vi "LV10_7.vi"() -> ()   [LabVIEW 2016]
uses:
  <vilib>/picture/picture.llb/Draw 8-Bit Pixmap.vi
  <vilib>/imath/engines/lvmath2/RunTimeEngine/BuiltInFunctions/randnormal/NIMS_randnormal(Str,I32).vi
  <vilib>/imathl/engines/lvmath/Functions/Error Handling/Create Error.vi
  <vilib>/imath/engines/lvmath2/RunTimeEngine/BuiltInFunctions/randnormal/NIMS_randnormal(I32,I32).vi
  <vilib>/imath/engines/lvmath2/RunTimeEngine/BuiltInFunctions/fft2d/NIMS_fft2d.vi
  <instcachedir>/0/NIMS_fft2d_01A33FFC48FF4786A19C9A8A715D9BC4.lvgen/NIMS_fft2d_01A33FFC48FF4786A19C9A8A715D9BC4_000.vi
  <vilib>/imath/engines/lvmath2/RunTimeEngine/BuiltInFunctions/abs/NIMS_abs(signed).vi
  <instcachedir>/0/NIMS_abs(signed)_C4FCB8E6058B49B797C7C8D53CA5F6EC.lvgen/NIMS_abs(signed)_C4FCB8E6058B49B797C7C8D53CA5F6EC_003.vi
  <vilib>/imath/engines/lvmath2/RunTimeEngine/BuiltInFunctions/findnz/NIMS_[1o]_findnz(GM).vi
  <instcachedir>/0/NIMS_[1o]_findnz(GM)_0B85F0C1FD7A4D70A7D15487030BA0C8.lvgen/NIMS_[1o]_findnz(GM)_0B85F0C1FD7A4D70A7D15487030BA0C8_004.vi
  <vilib>/imath/engines/lvmath2/RunTimeEngine/ErrorHandling/NIMS_Error From Error Code.vi
  <vilib>/imath/engines/lvmath2/RunTimeEngine/IndexReplace/NIMS M(S,S)=S.vi
  <instcachedir>/0/NIMS M(S,S)=S_98E40400474E4398B113AE20298B4F82.lvgen/NIMS M(S,S)=S_98E40400474E4398B113AE20298B4F82_002.vi
  <vilib>/imath/engines/lvmath2/RunTimeEngine/IndexRead/NIMS M(M).vi
  <instcachedir>/0/NIMS M(M)_EB00EBD471DD47B0915ED9997EB5A993.lvgen/NIMS M(M)_EB00EBD471DD47B0915ED9997EB5A993_004.vi
  <vilib>/imath/engines/lvmath2/RunTimeEngine/IndexReplace/NIMS M(M)=M.vi
  <instcachedir>/0/NIMS M(M)=M_D07272DCF1984374AF2B42254FCB82DF.lvgen/NIMS M(M)=M_D07272DCF1984374AF2B42254FCB82DF_003.vi
  <vilib>/imath/engines/lvmath2/RunTimeEngine/ErrorHandling/NIMS_Create Error From Enums.vi
  <vilib>/imath/engines/lvmath2/RunTimeEngine/BuiltInFunctions/norm/NIMS_norm(GV,DBL).vi
  <instcachedir>/0/NIMS_norm(GV,DBL)_1268AFF3C646412B8C6EA3CE75D09042.lvgen/NIMS_norm(GV,DBL)_1268AFF3C646412B8C6EA3CE75D09042_000.vi
  <vilib>/imath/engines/lvmath2/RunTimeEngine/BuiltInFunctions/length/NIMS_length(GV).vi
  <instcachedir>/0/NIMS_length(GV)_08A3D13377FD4E4B96F5795FBF3698FA.lvgen/NIMS_length(GV)_08A3D13377FD4E4B96F5795FBF3698FA_000.vi
  <vilib>/imath/engines/lvmath2/RunTimeEngine/BuiltInFunctions/mirrorh/NIMS_mirrorh(GRowV).vi
  <instcachedir>/0/NIMS_mirrorh(GRowV)_B6A8CC4EAFBA4F9A82A59460D67BDFF0.lvgen/NIMS_mirrorh(GRowV)_B6A8CC4EAFBA4F9A82A59460D67BDFF0_000.vi
  <vilib>/imath/engines/lvmath2/RunTimeEngine/RangeToken/NIMS_Range.vi
  <instcachedir>/0/NIMS_Range_A7C094595B484CA7AF10685B02D808ED.lvgen/NIMS_Range_A7C094595B484CA7AF10685B02D808ED_001.vi
  <vilib>/imath/engines/lvmath2/RunTimeEngine/ArithmeticOperatorToken/NIMS_ArithmeticOperator_times.vi
  <instcachedir>/0/NIMS_ArithmeticOperator_times_953B34F74CAC448FB707D816A29CC5F0.lvgen/NIMS_ArithmeticOperator_times_953B34F74CAC448FB707D816A29CC5F0_000.vi
  <vilib>/imath/engines/lvmath2/RunTimeEngine/NodeEndStatement/NIMS_NodeEndStatement_Output.vi
  <instcachedir>/0/NIMS_NodeEndStatement_Output_53EC0D466D134D7ABD903AC30B43404B.lvgen/NIMS_NodeEndStatement_Output_53EC0D466D134D7ABD903AC30B43404B_002.vi
  <instcachedir>/0/NIMS_NodeEndStatement_Output_53EC0D466D134D7ABD903AC30B43404B.lvgen/NIMS_NodeEndStatement_Output_53EC0D466D134D7ABD903AC30B43404B_011.vi
  <instcachedir>/0/NIMS_NodeEndStatement_Output_53EC0D466D134D7ABD903AC30B43404B.lvgen/NIMS_NodeEndStatement_Output_53EC0D466D134D7ABD903AC30B43404B_005.vi
  <vilib>/imath/engines/lvmath2/RunTimeEngine/ErrorHandling/NIMS_Finalize Error.vi
panel:
  in  "Threshold l for shrinking":dbl(slide)=0.01 scale=0.001..0.1
  out "Known pixel percentage":dbl=50.43
  out "Original image":picture
  out "Deteriorated image":picture
  in  "Missing pixel density":dbl(slide)=166.0 scale=100.0..200.0
  in  "Max iterations":i32(slide)=98 scale=1.0..500.0
  out "Iterations":i32(slide)=31 scale=-1.0..500.0
  out "Reconstructed image":picture
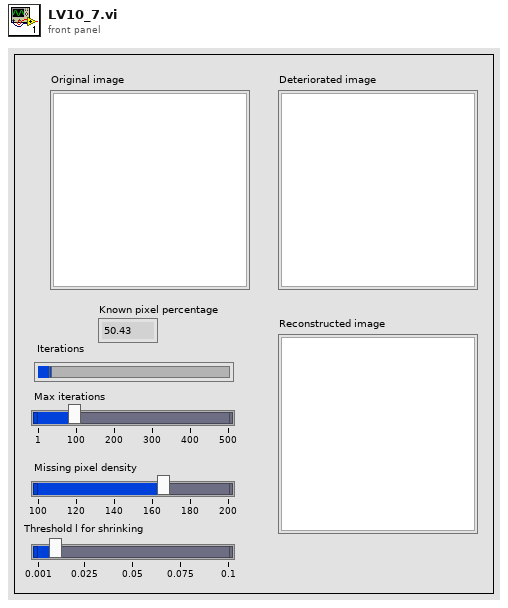
[diagram p1: front panel]
types:
  T1 = typedef "imagedata.ctl" = cluster{"image type":i32, "image depth":i32, "image":u8[], "mask":u8[], "colors":u32[], "Rectangle":cluster{"left":i16, "top":i16, "right":i16, "bottom":i16}}
  T2 = cluster{"ZLL1":dbl[][], "ZLL2":dbl[][], "ZLL3":dbl[][], "ZLH1":dbl[][], "ZLH2":dbl[][], "ZLH3":dbl[][], "ZHL1":dbl[][], "ZHL2":dbl[][], "ZHL3":dbl[][], "ZHH1":dbl[][], "ZHH2":dbl[][], "ZHH3":dbl[][]}
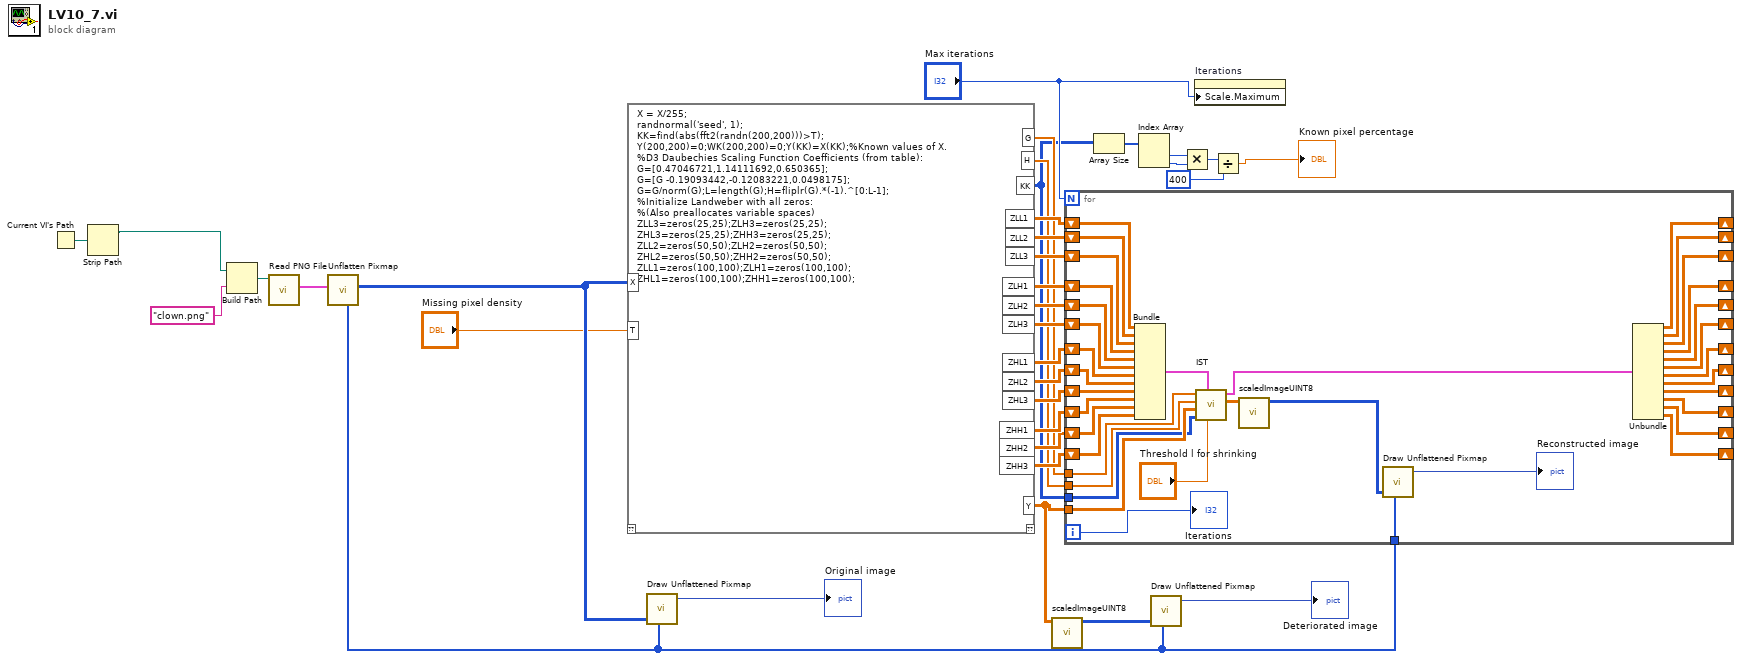
[diagram p0: block diagram]
diagram:
  n1 = Current VI's Path() -> (path=w34:path)
  n2 = Strip Path(path=w34) -> (stripped path=w1:path)  [unwired: 1 out]
  n3 = Build Path(base path=w1, name or relative path="clown.png") -> (appended path=w32:path)
  n4 = call <vilib>:"Read PNG File.vi"("path to PNG file"=w32) -> ("image data"=w31:T1)  [unwired: 8 in, 2 out]
  n5 = call <vilib>:"Unflatten Pixmap.vi"("image data"=w31) -> ("8-bit pixmap"=w29:u8[][], "colors"=w30:u32[])  [unwired: 4 in, 5 out]
  n6 = mathscript code="X = X/255;\nrandnormal('seed', 1);\nKK=find(abs(fft2(randn(200,200)))>T);\nY(200,200)=0;WK(200,200)=0;Y(KK)=X(KK);%Known values of X.\n%D3 Daubechies Scaling Function Coefficients (from table):\nG=[0.47046721,1.14111692,0.650365];\nG=[G -0.19093442,-0.12083221,0.0498175];\nG=G/norm(G);L=length(G);H=fliplr(G).*(-1).^[0:L-1];\n%Initialize Landweber with all zeros:\n%(Also preallocates variable spaces)\nZLL3=zeros(25,25);ZLH3=zeros(25,25);\nZHL3=zeros(25,25);ZHH3=zeros(25,25);\nZLL2=zeros(50,50);ZLH2=zeros(50,50);\nZHL2=zeros(50,50);ZHH2=zeros(50,50);\nZLL1=zeros(100,100);ZLH1=zeros(100,100);\nZHL1=zeros(100,100);ZHH1=zeros(100,100);"("X"=w29, "T"="Missing pixel density") -> ("ZHH1"=w19:dbl[][], "ZHH2"=w18:dbl[][], "ZHH3"=w17:dbl[][], "ZLL1"=w28:dbl[][], "ZLL2"=w27:dbl[][], "ZLH3"=w23:dbl[][], "ZLL3"=w26:dbl[][], "ZLH1"=w25:dbl[][], "ZLH2"=w24:dbl[][], "ZHL1"=w22:dbl[][], "ZHL2"=w21:dbl[][], "ZHL3"=w20:dbl[][], "G"=w16:dbl[], "H"=w15:dbl[], "KK"=w8:i32[][], "Y"=w9:dbl[][])  [unwired: 1 in, 1 out]
  n7 = call-poly <vilib>:"Draw Unflattened Pixmap.vi"("data"=w29, "color table"=w30) -> ("new picture"=→"Original image":picture)  [unwired: 7 in]
  n8 = call "scaledImageUINT8.vi"("double image"=w9) -> ("uint8 image"=w10:u8[][])  [unwired: 10 in]
  n9 = for {
    N: "Max iterations" -> [_]
    tunnel: w16 -> [w46]
    tunnel: w15 -> [w45]
    tunnel: w9 -> [w44]
    tunnel: w8 -> [w43]
    shift-right: [w58] -> _
    shift-left: w28 -> [w61]
    shift-right: [w57] -> _
    shift-left: w27 -> [w60]
    shift-right: [w56] -> _
    shift-left: w26 -> [w59]
    shift-right: [w55] -> _
    shift-left: w25 -> [w70]
    shift-right: [w54] -> _
    shift-left: w24 -> [w69]
    shift-right: [w53] -> _
    shift-left: w23 -> [w68]
    shift-right: [w52] -> _
    shift-left: w22 -> [w67]
    shift-right: [w51] -> _
    shift-left: w21 -> [w66]
    shift-right: [w50] -> _
    shift-left: w20 -> [w65]
    shift-right: [w49] -> _
    shift-left: w19 -> [w64]
    shift-right: [w48] -> _
    shift-left: w18 -> [w63]
    shift-right: [w47] -> _
    shift-left: w17 -> [w62]
    tunnel: w30 -> [w36]
    i -> [w37]
    n10 = Bundle("ZLL1"=w61, "ZLL2"=w60, "ZLL3"=w59, "ZLH1"=w70, "ZLH2"=w69, "ZLH3"=w68, "ZHL1"=w67, "ZHL2"=w66, "ZHL3"=w65, "ZHH1"=w64, "ZHH2"=w63, "ZHH3"=w62) -> (w41:T2)  [unwired: 1 in]
    n11 = call "IST.vi"("lambda"="Threshold l for shrinking", "Input"=w41, "KK"=w43, "Y"=w44, "H"=w45, "G"=w46) -> ("W"=w38:dbl[][], "output"=w42:T2)  [unwired: 4 in]
    n12 = call "scaledImageUINT8.vi"("double image"=w38) -> ("uint8 image"=w40:u8[][])  [unwired: 10 in]
    n13 = call-poly <vilib>:"Draw Unflattened Pixmap.vi"("data"=w40, "color table"=w36) -> ("new picture"=→"Reconstructed image":picture)  [unwired: 7 in]
    n14 = Unbundle(w42) -> ("ZLL1"=w58:dbl[][], "ZLL2"=w57:dbl[][], "ZLL3"=w56:dbl[][], "ZLH1"=w55:dbl[][], "ZLH2"=w54:dbl[][], "ZLH3"=w53:dbl[][], "ZHL1"=w52:dbl[][], "ZHL2"=w51:dbl[][], "ZHL3"=w50:dbl[][], "ZHH1"=w49:dbl[][], "ZHH2"=w48:dbl[][], "ZHH3"=w47:dbl[][])
    "Iterations" <- w37
  }
  n15 = Array Size(array=w8) -> (size(s)=w7:i32[])
  n16 = Index Array(array=w7) -> (element #1=w6:i32, element #2=w5:i32)  [unwired: 2 in]
  n17 = call-poly <vilib>:"Draw Unflattened Pixmap.vi"("data"=w10, "color table"=w30) -> ("new picture"=→"Deteriorated image":picture)  [unwired: 7 in]
  n18 = Multiply(x=w6, y=w5) -> (x*y=w4:i32)
  n19 = property on="Iterations" class="Slide (strict)"("Scale.Maximum"="Max iterations") -> ()  [unwired: 2 in, 2 out]
  n20 = Divide(x=w4, y=400) -> (x/y=→"Known pixel percentage":dbl)
